vi "Get Draw Error Clusters.vi"(8 "error in (no error)":errorcluster {"code" format="Error %.0f"}, 11 "VIDoc Parser In":refnum<class "VIDoc Parser.lvclass">) -> (0 "error out":errorcluster {"code" format="Error %.0f"}, 2 "Option":T1, 3 "VIDoc Parser Out":refnum<class "VIDoc Parser.lvclass">)   [LabVIEW 2023, in "VIDoc Parsing.lvlib" / "VIDoc Parser.lvclass"]
uses:
  VIDoc Parser.lvclass
  Settings/Parser Settings/Draw Option Enum.ctl
  Settings/Parser Settings/Parser Settings.lvclass
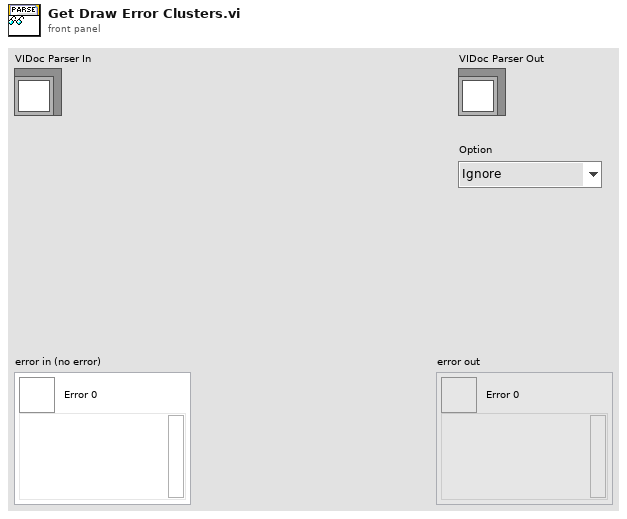
[diagram p1: front panel]
types:
  T1 = typedef "VIDoc Parsing.lvlib/Parser Settings.lvclass/Draw Option Enum.ctl" = enum16{"Ignore", "Draw", "Draw + Contents"}
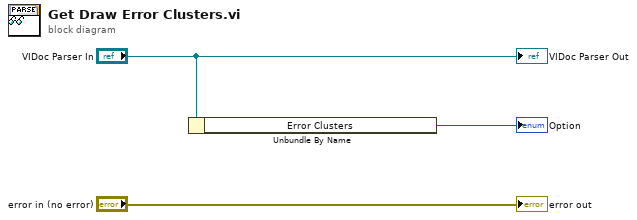
[diagram p0: block diagram]
diagram:
  n1 = Unbundle By Name("VIDoc Parser In") -> ("Error Clusters"=→"Option":T1)
  "error out" <- "error in (no error)"
  "VIDoc Parser Out" <- "VIDoc Parser In"
